vi "stopAllANDWait.vi"(8 "error in (no error)":errorcluster, 11 "Tapedrive_ESP301 in":refnum<class "Tapedrive_ESP301.lvclass">) -> (0 "error out":errorcluster, 3 "Tapedrive_ESP301 out":refnum<class "Tapedrive_ESP301.lvclass">)   [LabVIEW 2013, in "Tapedrive_ESP301.lvclass"]
uses:
  Tapedrive_ESP301.lvclass
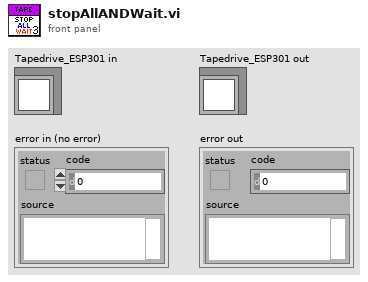
[diagram p1: front panel]
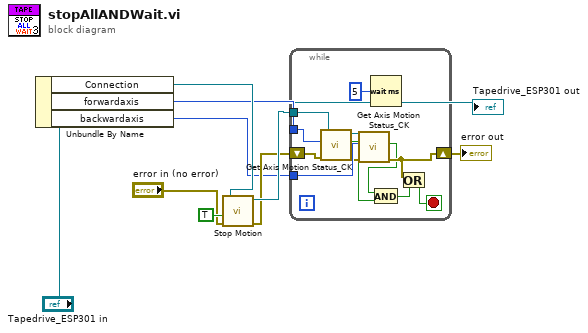
[diagram p0: block diagram]
diagram:
  n1 = Unbundle By Name("Tapedrive_ESP301 in") -> ("Connection"=w6:refnum<visa-resource-name>, "forwardaxis"=w2:i16, "backwardaxis"=w3:i16)
  n2 = call <instrlib>:"Stop Motion.vi"("error in (no error)"="error in (no error)", "Stop all axes (F)"=TRUE, "VISA resource name"=w6) -> ("error out"=w5:errorcluster, "VISA resource name out"=w7:refnum<visa-resource-name>)  [unwired: 3 in]
  n3 = while {
    tunnel: w2 -> [w21]
    tunnel: w7 -> [w20]
    tunnel: w3 -> [w18]
    shift-right: [w17] -> w9
    shift-left: w5 -> [w15]
    stop <- w11 stop-if-true
    n4 = call "Get Axis Motion Status_CK.vi"("error in (no error)"=w15, "Axis (1)"=w21, "VISA resource name"=w20) -> ("error out"=w16:errorcluster, "Motion Done"=w13:bool, "VISA resource name out"=w19:refnum<visa-resource-name>)  [unwired: 2 in]
    n5 = call "Get Axis Motion Status_CK.vi"("error in (no error)"=w16, "Axis (1)"=w18, "VISA resource name"=w19) -> ("error out"=w17:errorcluster, "Motion Done"=w14:bool)  [unwired: 2 in, 1 out]
    n6 = Wait (ms)(milliseconds to wait=u32 5) -> ()  [unwired: 1 out]
    n7 = And(x=w14, y=w13) -> (x .and. y?=w12:bool)
    n8 = Or(x=w17, y=w12) -> (x .or. y?=w11:bool)
  }
  "error out" <- w9
  "Tapedrive_ESP301 out" <- "Tapedrive_ESP301 in"
